vi "dfd_Format Number (Options).vi"(5 "format string":string, 6 "Is Lower Coefficient?":bool, 7 "Is Higher Coeffiecient?":bool, 11 "Coefficient":dbl) -> (3 "String Coefficient":string)   [LabVIEW 2017, in "NI_DigFilter_Process.lvlib"]
uses:
  <vilib>/addons/Digital Filter Design/NI_DigFilter_Process.lvlib
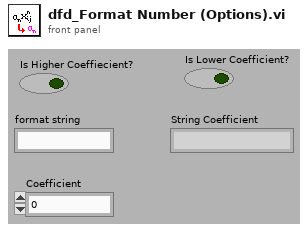
[diagram p1: front panel]
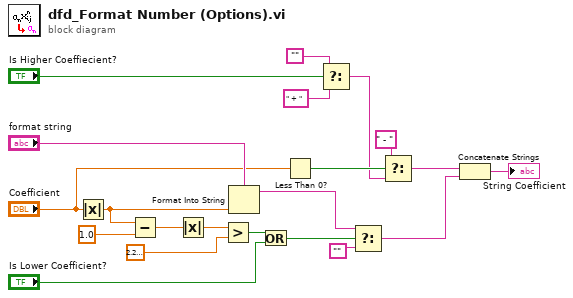
[diagram p0: block diagram]
diagram:
  n1 = Absolute Value(x="Coefficient") -> (abs(x)=w6:dbl)
  n2 = Subtract(x=w6, y=1.0) -> (x-y=w3:dbl)
  n3 = Absolute Value(x=w3) -> (abs(x)=w2:dbl)
  n4 = Greater?(x=w2, y=2.220446049250313e-16) -> (0:w4:bool)
  n5 = Format Into String(format string="format string", w6) -> (resulting string=w11:string)  [unwired: 2 in, 1 out]
  n6 = Or(x=w4, y="Is Lower Coefficient?") -> (x .or. y?=w9:bool)
  n7 = Less Than 0?(x="Coefficient") -> (x < 0?=w20:bool)
  n8 = Select(t="", s="Is Higher Coeffiecient?", f=" + " ("string")) -> (s? t:f=w15:string)
  n9 = Select(t=w11, s=w9, f="") -> (s? t:f=w10:string)
  n10 = Select(t=" - " ("string"), s=w20, f=w15) -> (s? t:f=w14:string)
  n11 = Concatenate Strings(w14, w10) -> (→"String Coefficient":string)
